vi "Write Input.vi"(8 "error in (no error)":errorcluster, 10 "External Reference":variant, 11 "Command with External Ref in":refnum<class "Command with Input.lvclass">) -> (0 "error out":errorcluster, 3 "Command with External Ref out":refnum<class "Command with Input.lvclass">)   [LabVIEW 2017, in "Command Handler.lvlib" / "Command with Input.lvclass"]
uses:
  Command with Input.lvclass
  Command with Input.lvclass/Command with Input.ctl
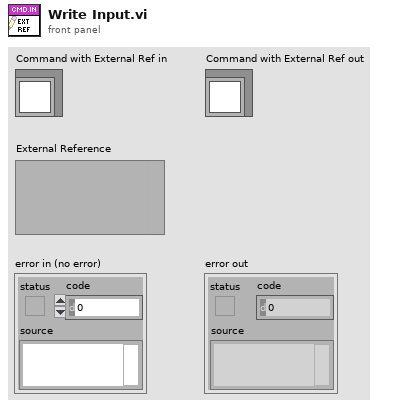
[diagram p1: front panel]
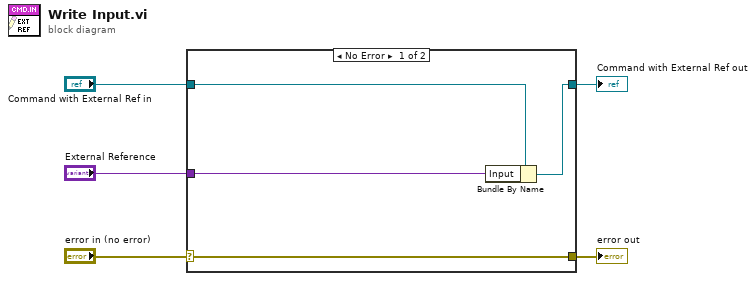
[diagram p0: block diagram]
diagram:
  n1 = case shown="No Error" "error in (no error)" {
    selector: "error in (no error)" -> [w9 w10]
    tunnel: [w9 w10] -> w4
    tunnel: [w7 w11] -> w2
    tunnel: "Command with External Ref in" -> [w8 w11]
    tunnel: "External Reference" -> [w6 _]
    frame No Error {
      n2 = Bundle By Name(cluster=w8, "Input"=w6) -> (w7:refnum<class "Command with Input.lvclass">)
    }
    frame Error {
    }
  }
  "error out" <- w4
  "Command with External Ref out" <- w2
